vi "Instantiate Function [On Syntax].vi"(0 "function manager in":refnum<class "function manager.lvclass">, 5 "Function String":string, 11 "error in (no error)":errorcluster) -> (4 "function manager out":refnum<class "function manager.lvclass">, 6 "function obj":refnum<class "functionbase.lvclass">, 8 "Valid Syntax?":bool, 15 "error out":errorcluster)   [LabVIEW 2016, in "function manager.lvclass"]
uses:
  function manager.lvclass
  functionsbase/functionbase.lvclass
  function manager.lvclass/function manager.ctl
  functionsbase/functionbase.lvclass/functionbase.ctl
  functionsbase/properties/Write Func Syntax.vi
  functionsbase/properties/Write Func Full String.vi
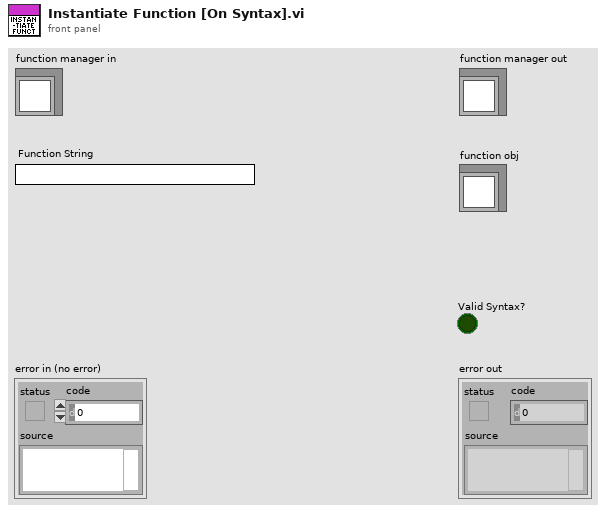
[diagram p1: front panel]
types:
  T1 = typedef "Syntax Format.ctl" = cluster{"Syntax":string, "Variable#":T2}
  T2 = typedef "Variable#.ctl" = enum16{"Zero", "One", "Two", "Three", "Four", "Five"}
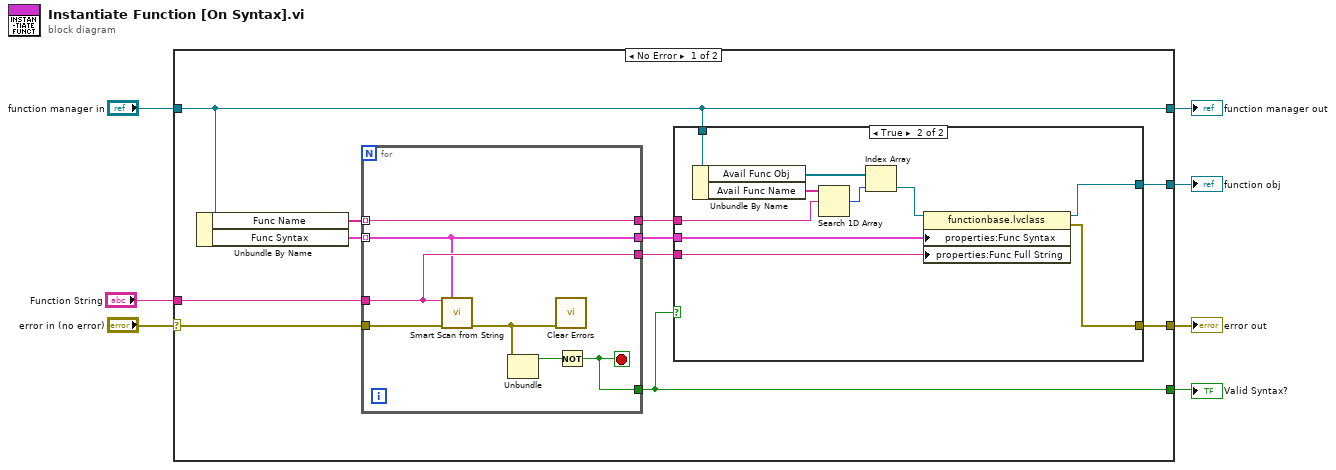
[diagram p0: block diagram]
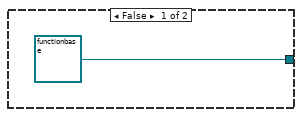
[diagram p2: hidden frame]
diagram:
  n1 = case shown="No Error" "error in (no error)" {
    selector: "error in (no error)" -> [w15 w38]
    tunnel: [w10 w38] -> w6
    tunnel: [w14 w37] -> w4
    tunnel: "function manager in" -> [w14 w37]
    tunnel: "Function String" -> [w18 _]
    tunnel: [w8 _] -> w2
    tunnel: [w9 _] -> w1
    frame No Error {
      n2 = Unbundle By Name(w14) -> ("Func Name"=w16:string[], "Func Syntax"=w17:T1[])
      n3 = for {
        tunnel: w18 -> [w31]
        tunnel: w17 -> [w30] mode=indexing
        tunnel: w16 -> [w34] mode=indexing
        tunnel: w15 -> [w33]
        tunnel: [w35] -> w8
        tunnel: [w34] -> w13
        tunnel: [w30] -> w12
        tunnel: [w31] -> w11
        stop <- w35 stop-if-true
        n4 = call "Smart Scan from String.vi"("initial string"=w31, "Syntax Format"=w30, "error in"=w33) -> ("error out"=w32:errorcluster)  [unwired: 10 in, 2 out]
        n5 = Unbundle(w32) -> ("status"=w36:bool)  [unwired: 2 out]
        n6 = call <vilib>:"Clear Errors.vi"("error in (no error)"=w32) -> ()  [unwired: 5 in, 2 out]
        n7 = Not(x=w36) -> (.not. x?=w35:bool)
      }
      n8 = case shown="True" w8 {
        tunnel: w14 -> [_ w29]
        tunnel: w13 -> [_ w27]
        tunnel: w12 -> [_ w20]
        tunnel: w11 -> [_ w23]
        tunnel: [_ w22] -> w10
        tunnel: [refnum<class "functionbase.lvclass"> refnum ("functionbase.lvclass") w21] -> w9
        frame False {
        }
        frame True {
          n9 = Unbundle By Name(w29) -> ("Avail Func Obj"=w26:refnum<class "functionbase.lvclass">[], "Avail Func Name"=w28:string[])
          n10 = Search 1D Array(1D array=w28, element=w27) -> (index of element=w25:i32)  [unwired: 1 in]
          n11 = Index Array(array=w26, index=w25) -> (element=w24:refnum<class "functionbase.lvclass">)
          n12 = property class="functionbase.lvclass"(reference=w24, "properties:Func Syntax"=w20, "properties:Func Full String"=w23) -> (reference out=w21:refnum<class "functionbase.lvclass">, error out=w22:errorcluster)  [unwired: 1 in]
        }
      }
    }
    frame Error {
    }
  }
  "error out" <- w6
  "function manager out" <- w4
  "Valid Syntax?" <- w2
  "function obj" <- w1
